vi "Failure.vi"(7 "Name":string="Failure", 11 "Node In":refnum<class "abs_Node.lvclass">) -> (3 "Node":refnum<class "abs_Node.lvclass">)   [LabVIEW 2021, in "BT.lvlib"]
uses:
  BT.lvlib
  Support/abs_Node/abs_Node.lvclass
  Support/Failure/Failure.lvclass
  C:/Users/Tim/Documents/GitHub/LV_Behaviour_Tree/Source/Support/abs_Decorator/abs_Decorator.lvclass
  C:/Program Files (x86)/National Instruments/LabVIEW 2021/vi.lib/TSA/Abstract Data Classes/Abs_Types/Type/Abs_Type.lvclass
  C:/Users/Tim/Documents/GitHub/LV_Behaviour_Tree/Source/Support/abs_Node/abs_Node.lvclass
  Support/abs_Decorator/abs_Decorator.lvclass/abs_Decorator.ctl
  <vilib>/TSA/Abstract Data Classes/Abs_Types/Type/Abs_Type.lvclass/Abs_Type.ctl
  Support/abs_Decorator/Properties/Write Node.vi
  <vilib>/TSA/Abstract Data Classes/Abs_Types/Type/Properties/Write Name.vi
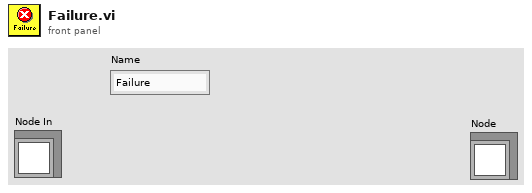
[diagram p1: front panel]
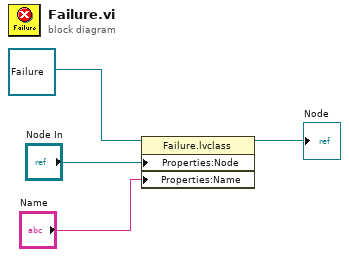
[diagram p0: block diagram]
diagram:
  n1 = property class="Failure.lvclass"(reference=refnum<class "Failure.lvclass"> refnum ("BT.lvlib:Failure.lvclass"), "Properties:Node"="Node In", "Properties:Name"="Name") -> (reference out=→"Node":refnum<class "Failure.lvclass">)  [unwired: 1 in, 1 out]
